vi "ResetChannelVI.vi"(0 "Angelsample":dbl[](array[numeric]), 1 "Angel":bool[](array[boolean]), 2 "dt":dbl, 5 "Torquesample":dbl[](array[numeric]), 7 "Torque":bool[](array[boolean]), 9 "ResetAngel":dbl[](array[numeric]), 11 "ResetTorqueCommand":dbl[](array[numeric]), 12 "ChannelSetArray":T1[](array[typedef]) {"Enable" items=["不使能", "使能"]; "Wave" items=["0指令", "正弦波", "方波", "三角波", "常值", "波形数据", "白噪声", "正弦扫频", "梯度加载", "VMIC"]; "ChannelType" items=["标准波形跟踪"=1, "扫频测试"=2, "消除多余力"=3, "梯度加载"=4, "载荷谱跟踪"=5, "模拟输入跟踪"=9]; "ChannelStatus" items=["通道关", "位置通道", "加载通道"]}, 13 "AxisForceSample":dbl[](array[numeric])) -> (4 "ControlOutput":dbl[](array[numeric]), 6 "resetAngel 2":dbl[](array[numeric]), 10 "ResetTorque 2":dbl[](array[numeric]), 15 "Commandout":dbl[](array[numeric]))   [LabVIEW 2020]
uses:
  ChannelCommand.ctl
  Control 1.ctl
  WaveType.ctl
  MoterEnable.ctl
  <vilib>/addons/control/pid/pid.llb/PID (DBL Array).vi
  <vilib>/addons/control/pid/NI_PID_pid.lvlib
panel:
  out "PXI6738DATask 2":refnum<k21>
  out "PXI6738DATask":refnum<k21>
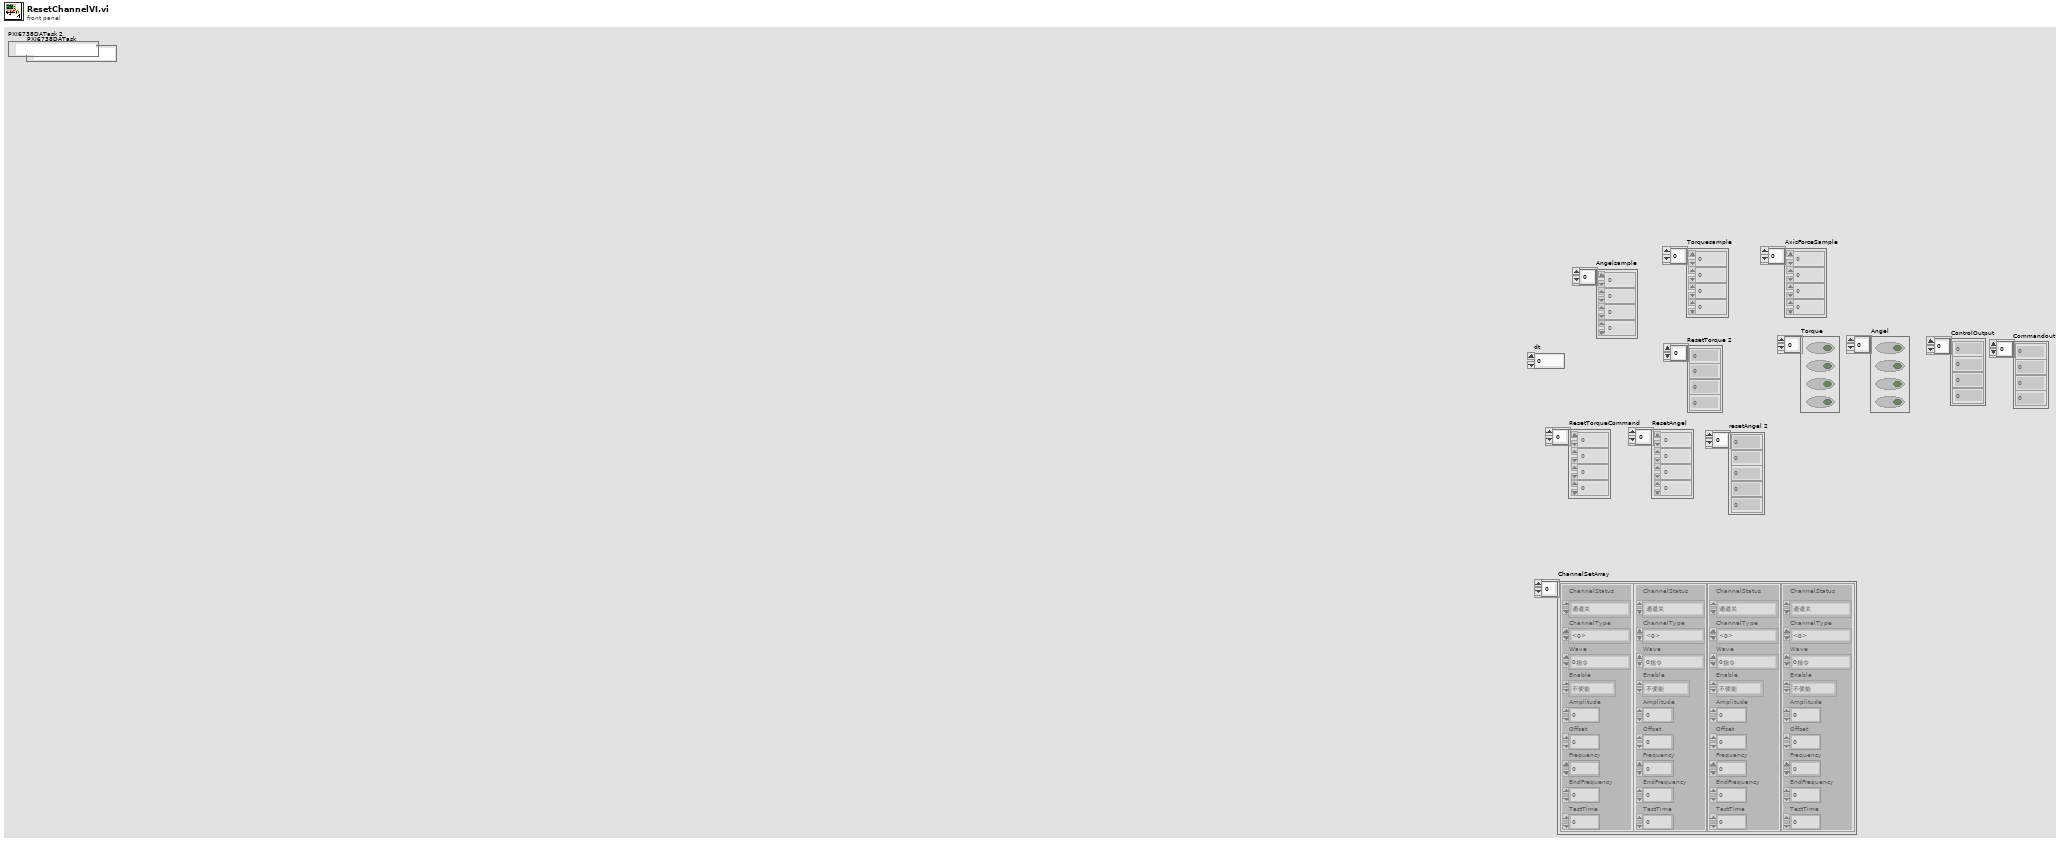
[diagram p1: front panel]
types:
  T1 = typedef "ChannelCommand.ctl" = cluster{"ChannelStatus":T2, "ChannelType":i32, "Wave":T3, "Enable":T4, "Amplitude":dbl, "Offset":dbl, "Frequency":dbl, "EndFrequency":dbl, "TestTime":dbl}
  T2 = typedef "Control 1.ctl" = i32
  T3 = typedef "WaveType.ctl" = i32
  T4 = typedef "MoterEnable.ctl" = u16
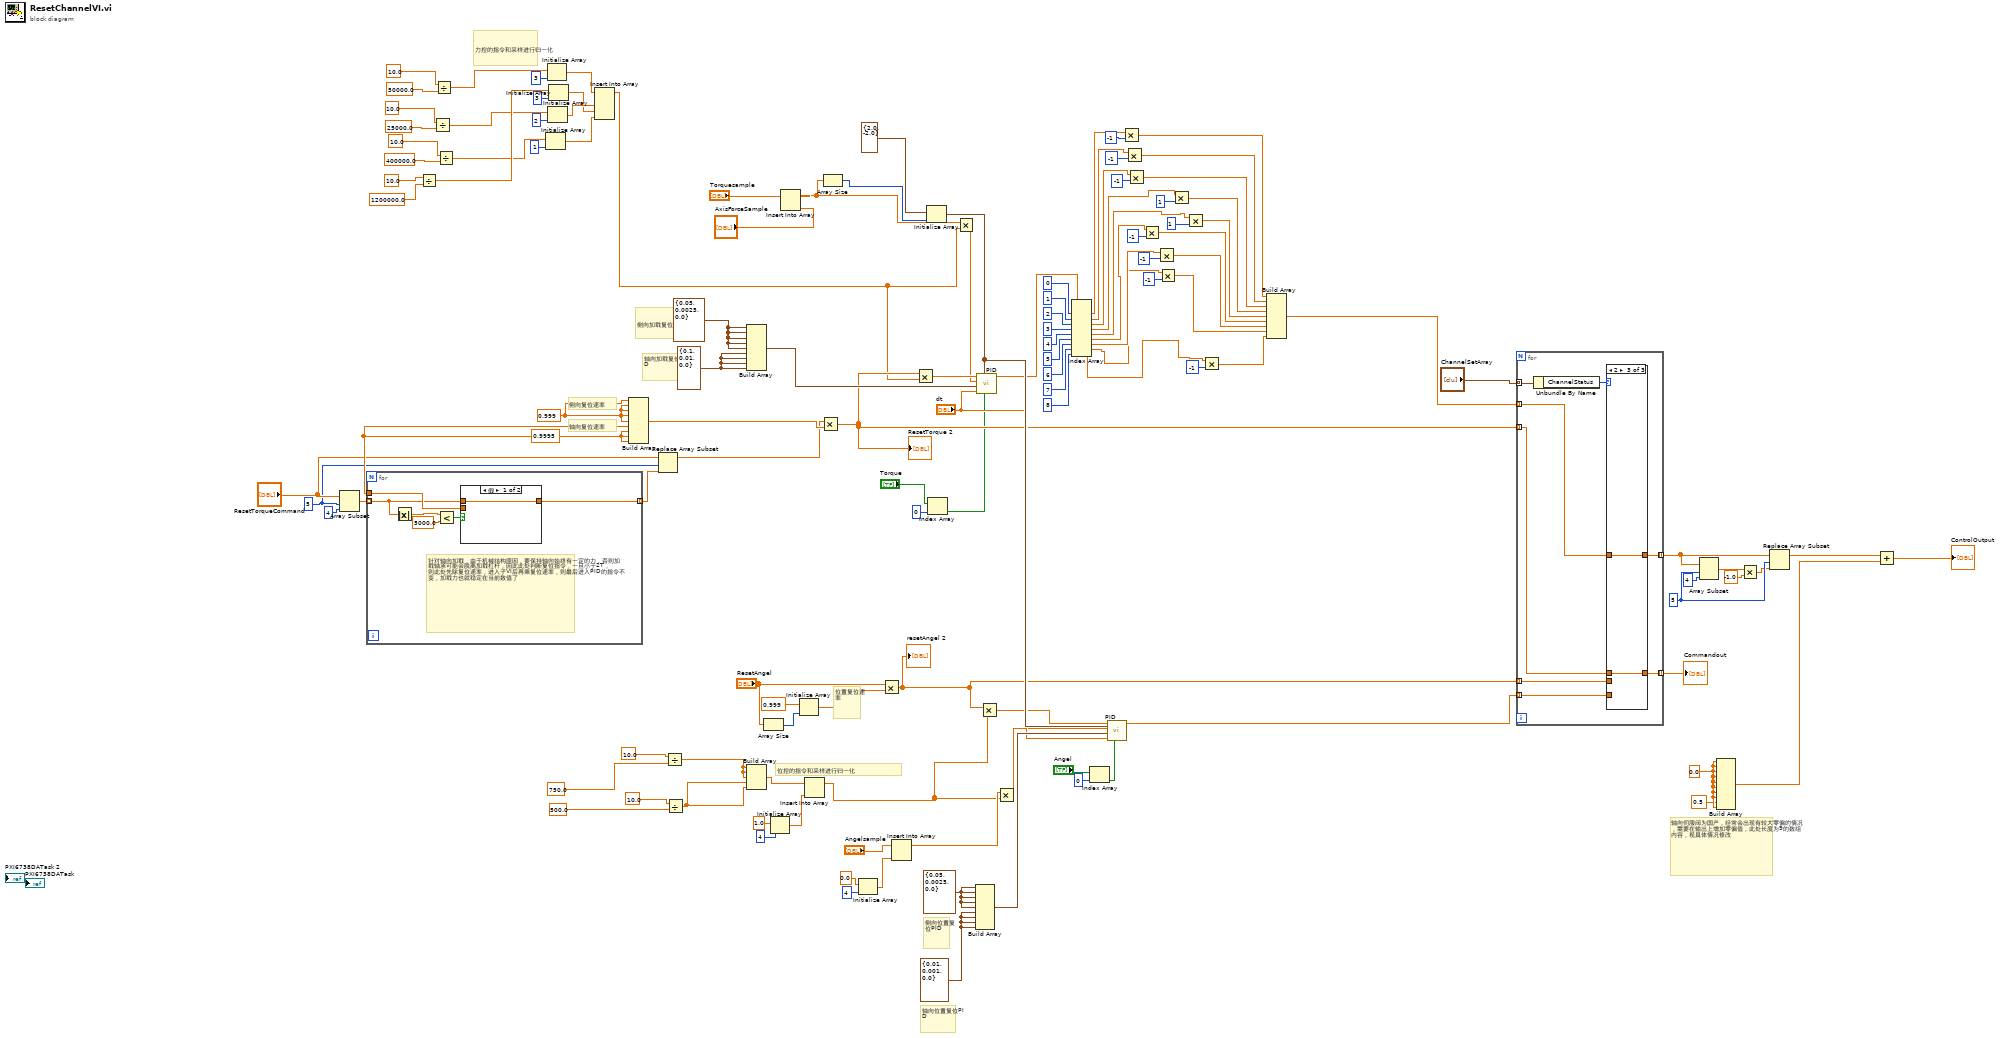
[diagram p0: block diagram]
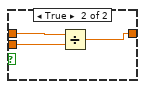
[diagram p2: hidden frame]
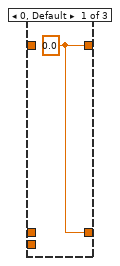
[diagram p3: hidden frame]
diagram:
  w76 = 5 ("索引")
  w107 = cluster{dbl, dbl, dbl} {0.05, 0.0025, 0.0} ("簇")
  w106 = cluster{dbl, dbl, dbl} {0.01, 0.001, 0.0} ("簇")
  w111 = 0.999
  w112 = 0.0
  w119 = 5 ("索引")
  w78 = 0.9995
  w127 = cluster{dbl, dbl, dbl} {0.05, 0.0025, 0.0} ("簇")
  w126 = cluster{dbl, dbl, dbl} {0.1, 0.01, 0.0} ("簇")
  # "位置复位速率"
  # "位控的指令和采样进行归一化"
  # "力控的指令和采样进行归一化"
  # "轴向位置复位PID"
  # "侧向位置复位PID"
  # "侧向复位速率"
  # "轴向伺服阀为国产，经常会出现有较大零偏的情况，需要在输出上增加零偏值，此处长度为9的数组内容，视具体情况修改"
  # "轴向复位速率"
  # "轴向加载复位PID"
  # "侧向加载复位PID"
  n1 = Array Subset(array="ResetTorqueCommand", index=w76, length=4 ("长度")) -> (w79:dbl[])
  n2 = for {
    tunnel: w79 -> [w129] mode=indexing
    tunnel: w78 -> [w131]
    tunnel: [w130] -> w75 mode=indexing
    # "针对轴向加载，由于机械结构原因，要保持轴向始终有一定的力，否则加载轴承可能会脱离加载杠杆，因此此处判断复位指令，一旦小于2T，\n则此处先除复位速率，进入子VI后再乘复位速率，则最后进入PID的指令不变，加载力也就稳定在当前数值了"
    n3 = Absolute Value(x=w129) -> (abs(x)=w128:dbl)
    n4 = Less?(x=w128, y=5000.0) -> (x < y?=w132:bool)
    n5 = case shown="假" w132 {
      tunnel: w129 -> [w134 w137]
      tunnel: [w134 w136] -> w130
      tunnel: w131 -> [_ w135]
      frame False {
      }
      frame True {
        n6 = Divide(x=w137, y=w135) -> (x/y=w136:dbl)
      }
    }
  }
  n7 = Divide(x=10.0 ("元素"), y=1200000.0) -> (x/y=w71:dbl)
  n8 = Divide(x=10.0 ("元素"), y=25000.0) -> (x/y=w56:dbl)
  n9 = Divide(x=10.0 ("元素"), y=50000.0) -> (x/y=w70:dbl)
  n10 = Divide(x=10.0 ("元素"), y=400000.0) -> (x/y=w57:dbl)
  n11 = Initialize Array(w57, 1 ("维数大小")) -> (w54:dbl[])
  n12 = Initialize Array(w70, 3 ("维数大小")) -> (w55:dbl[])
  n13 = Initialize Array(w56, 2 ("维数大小")) -> (w53:dbl[])
  n14 = Initialize Array(w71, 3 ("维数大小")) -> (w52:dbl[])
  n15 = Insert Into Array(array=w55, new element #1=w53, new element #2=w52, new element #3=w54) -> (w51:dbl[])  [unwired: 1 in]
  n16 = Build Array(w111, w111, w111, w111, w111, w78, w78, w78, w78) -> (w110:dbl[])
  n17 = Replace Array Subset(array="ResetTorqueCommand", new element=w75, index=w76) -> (w74:dbl[])
  n18 = Divide(x=10.0 ("元素"), y=750.0) -> (x/y=w46:dbl)
  n19 = Divide(x=10.0 ("元素"), y=500.0) -> (x/y=w45:dbl)
  n20 = Build Array(w127, w127, w127, w127, w127, w126, w126, w126, w126) -> (w109:cluster{dbl, dbl, dbl}[])
  n21 = Build Array(w46, w46, w46, w45, w45) -> (w44:dbl[])
  n22 = Array Size(array="ResetAngel") -> (size(s)=w97:i32)
  n23 = Initialize Array(1.0 ("元素"), 4 ("维数大小")) -> (w41:dbl[])
  n24 = Insert Into Array(array="Torquesample", new element="AxisForceSample") -> (w73:dbl[])  [unwired: 1 in]
  n25 = Initialize Array(0.999 ("元素"), w97) -> (w99:dbl[])
  n26 = Insert Into Array(array=w44, new element=w41) -> (w40:dbl[])  [unwired: 1 in]
  n27 = Multiply(x=w74, y=w110) -> (x*y=w87:dbl[])
  "ResetTorque 2" <- w87
  n28 = Array Size(array=w73) -> (size(s)=w72:i32)
  n29 = Initialize Array(0.0 ("元素"), 4 ("维数大小")) -> (w121:dbl[])
  n30 = Multiply(x="ResetAngel", y=w99) -> (x*y=w88:dbl[])
  "resetAngel 2" <- w88
  n31 = Insert Into Array(array="Angelsample", new element=w121) -> (w90:dbl[])  [unwired: 1 in]
  n32 = Multiply(x=w87, y=w51) -> (x*y=w94:dbl[])
  n33 = Initialize Array(cluster{"output high":dbl, "output low":dbl} {"output high"=2.0, "output low"=-2.0} ("output range"), w72) -> (w104:cluster{"output high":dbl, "output low":dbl}[])
  n34 = Index Array(array="Torque", index=0 ("索引")) -> (element=w83:bool)
  n35 = Multiply(x=w73, y=w51) -> (x*y=w93:dbl[])
  n36 = Build Array(w107, w107, w107, w107, w107, w106, w106, w106, w106) -> (w105:cluster{dbl, dbl, dbl}[])
  n37 = call-poly <vilib>:"PID.vi"("reinitialize? (F)"=w83, "output range"=w104, "dt (s)"="dt", "PID gains"=w109, "process variable"=w93, "setpoint"=w94) -> ("output"=w30:dbl[])  [unwired: 4 in, 1 out]
  n38 = Multiply(x=w88, y=w40) -> (x*y=w91:dbl[])
  n39 = Multiply(x=w90, y=w40) -> (x*y=w89:dbl[])
  n40 = Index Array(array=w30, index #1=0 ("索引"), index #2=1 ("索引"), index #3=2 ("索引"), index #4=3 ("索引"), index #5=4 ("索引"), index #6=5 ("索引"), index #7=6 ("索引"), index #8=7 ("索引"), index #9=8 ("索引")) -> (element #1=w29:dbl, element #2=w24:dbl, element #3=w21:dbl, element #4=w6:dbl, element #5=w5:dbl, element #6=w16:dbl, element #7=w13:dbl, element #8=w12:dbl, element #9=w2:dbl)
  n41 = Index Array(array="Angel", index=0 ("索引")) -> (element=w80:bool)
  n42 = call-poly <vilib>:"PID.vi"("reinitialize? (F)"=w80, "output range"=w104, "dt (s)"="dt", "PID gains"=w105, "process variable"=w89, "setpoint"=w91) -> ("output"=w102:dbl[])  [unwired: 4 in, 1 out]
  n43 = Multiply(x=w29, y=-1) -> (x*y=w27:dbl)
  n44 = Multiply(x=w24, y=-1) -> (x*y=w25:dbl)
  n45 = Multiply(x=w21, y=-1) -> (x*y=w22:dbl)
  n46 = Multiply(x=w16, y=-1) -> (x*y=w15:dbl)
  n47 = Multiply(x=w13, y=-1) -> (x*y=w14:dbl)
  n48 = Multiply(x=w12, y=-1) -> (x*y=w11:dbl)
  n49 = Multiply(x=w6, y=1) -> (x*y=w8:dbl)
  n50 = Multiply(x=w5, y=1) -> (x*y=w7:dbl)
  n51 = Multiply(x=w2, y=-1) -> (x*y=w1:dbl)
  n52 = Build Array(w27, w25, w22, w8, w7, w15, w14, w11, w1) -> (w20:dbl[])
  n53 = for {
    tunnel: "ChannelSetArray" -> [w145] mode=indexing
    tunnel: w20 -> [w144] mode=indexing
    tunnel: w102 -> [w143] mode=indexing
    tunnel: [w141] -> w101 mode=indexing
    tunnel: w88 -> [w140] mode=indexing
    tunnel: w87 -> [w139] mode=indexing
    tunnel: [w138] -> w86 mode=indexing
    n54 = Unbundle By Name(w145) -> ("ChannelStatus"=w142:T2)
    n55 = case shown="2" w142 {
      tunnel: w144 -> [_ _ w150]
      tunnel: w143 -> [_ w148 _]
      tunnel: [w146 w148 w150] -> w141
      tunnel: w140 -> [_ w147 _]
      tunnel: [w146 w147 w149] -> w138
      tunnel: w139 -> [_ _ w149]
      frame 0, Default {
        w146 = 0.0
      }
      frame 1 {
      }
      frame 2 {
      }
    }
  }
  "Commandout" <- w86
  n56 = Array Subset(array=w101, index=w119, length=4 ("长度")) -> (w100:dbl[])
  n57 = Build Array(w112, w112, w112, w112, w112, w112, w112, w112, w112, 0.5) -> (w115:dbl[])
  n58 = Multiply(x=w100, y=-1.0) -> (x*y=w118:dbl[])
  n59 = Replace Array Subset(array=w101, new element=w118, index=w119) -> (w114:dbl[])
  n60 = Add(x=w114, y=w115) -> (x+y=→"ControlOutput":dbl[])
